vi "001_while_loop_inside_stop_btn.vi"() -> ()   [LabVIEW 2024]
panel:
  in  "stop":bool
  out "Light":bool
  in  "Switch":bool
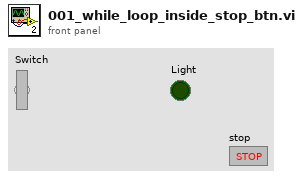
[diagram p1: front panel]
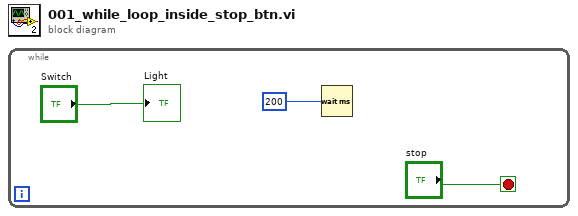
[diagram p0: block diagram]
diagram:
  n1 = while {
    stop <- "stop" stop-if-true
    n2 = Wait (ms)(milliseconds to wait=u32 200 ("millisecond timer value")) -> ()  [unwired: 1 out]
    "Light" <- "Switch"
  }
